vi "ArmXYZToR-L-E.vi"(9 "Z":dbl, 10 "Y":dbl, 11 "X":dbl) -> (1 "Extend":dbl, 2 "Lift":dbl, 3 "Rotate":dbl)   [LabVIEW 2020]
doc: "Take X, Y and Z values and output, with complicated math, Rotate, Lift, Extend values to get to that point\n\nInputs:\n--X--Double\n--Y--Double\n--Z--Double\n\nOutputs:\n--Rotate--Double--Degrees\n--Lift--Double--Degrees\n--Extend--Double--Inches"
uses:
  <vilib>/Rock Robotics/WPI/ThirdParty/JAS_Junk/TrajLib/Trajectory_Library.lvlib
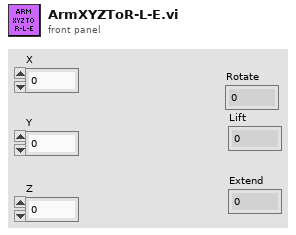
[diagram p1: front panel]
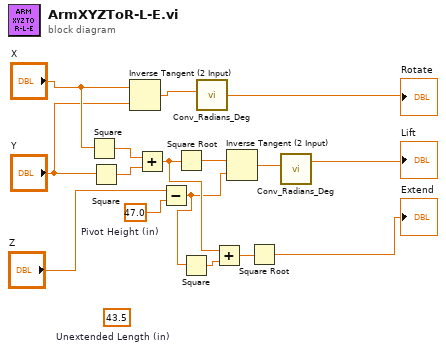
[diagram p0: block diagram]
diagram:
  (unwired) 43.5  # Unextended Length (in)
  w8 = 47.0  # Pivot Height (in)
  n1 = Square(x="X") -> (x^2=w12:dbl)
  n2 = Square(x="Y") -> (x^2=w11:dbl)
  n3 = Inverse Tangent (2 Input)(1:"Y", 2:"X") -> (0:w16:dbl)
  n4 = Add(x=w12, y=w11) -> (x+y=w5:dbl)
  n5 = Subtract(x="Z", y=w8) -> (x-y=w4:dbl)
  n6 = Square Root(x=w5) -> (sqrt(x)=w10:dbl)
  n7 = Square(x=w4) -> (x^2=w3:dbl)
  n8 = call <vilib>:"Conv_Radians_Deg.vi"("Radians"=w16) -> ("Degrees"=→"Rotate":dbl)  [unwired: 10 in]
  n9 = Add(x=w5, y=w3) -> (x+y=w2:dbl)
  n10 = Inverse Tangent (2 Input)(1:w4, 2:w10) -> (0:w7:dbl)
  n11 = Square Root(x=w2) -> (sqrt(x)=→"Extend":dbl)
  n12 = call <vilib>:"Conv_Radians_Deg.vi"("Radians"=w7) -> ("Degrees"=→"Lift":dbl)  [unwired: 10 in]
